vi "same.vi"(8 "error in (no error)":errorcluster, 10 "Name":string, 11 "Goal in":refnum<class "Goal.lvclass">) -> (0 "error out":errorcluster, 2 "Equals?":bool, 3 "Goal out":refnum<class "Goal.lvclass">)   [LabVIEW 2020, in "Goal.lvclass"]
uses:
  Goal.lvclass
  Goal.lvclass/Goal.ctl
  Category/Category.lvclass
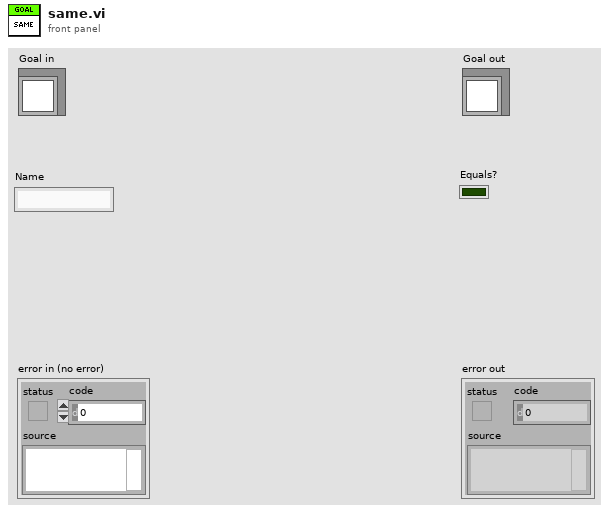
[diagram p1: front panel]
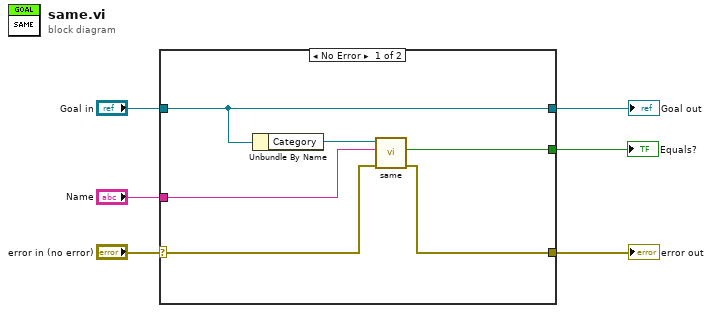
[diagram p0: block diagram]
diagram:
  n1 = case shown="No Error" "error in (no error)" {
    selector: "error in (no error)" -> [w10 w14]
    tunnel: [w9 w14] -> w5
    tunnel: [w12 w13] -> w3
    tunnel: "Goal in" -> [w12 w13]
    tunnel: [w8 _] -> w2
    tunnel: "Name" -> [w7 _]
    frame No Error {
      n2 = Unbundle By Name(w12) -> ("Category"=w11:refnum<class "Category.lvclass">)
      n3 = call "same.vi"("error in (no error)"=w10, "Name"=w7, "Category in"=w11) -> ("error out"=w9:errorcluster, "Equals?"=w8:bool)  [unwired: 6 in, 1 out]
    }
    frame Error {
    }
  }
  "error out" <- w5
  "Goal out" <- w3
  "Equals?" <- w2
